vi "TopLevel.vi"() -> ()   [LabVIEW 2020]
uses:
  <vilib>/Averna/ProligentResultProcessor/ProligentResultProcessor.lvlibp/Datawarehouse/Datawarehouse.lvclass
panel:
  out "Passed":bool
  out "error out":errorcluster
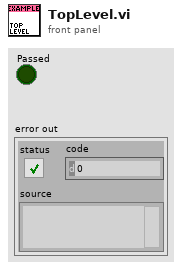
[diagram p1: front panel]
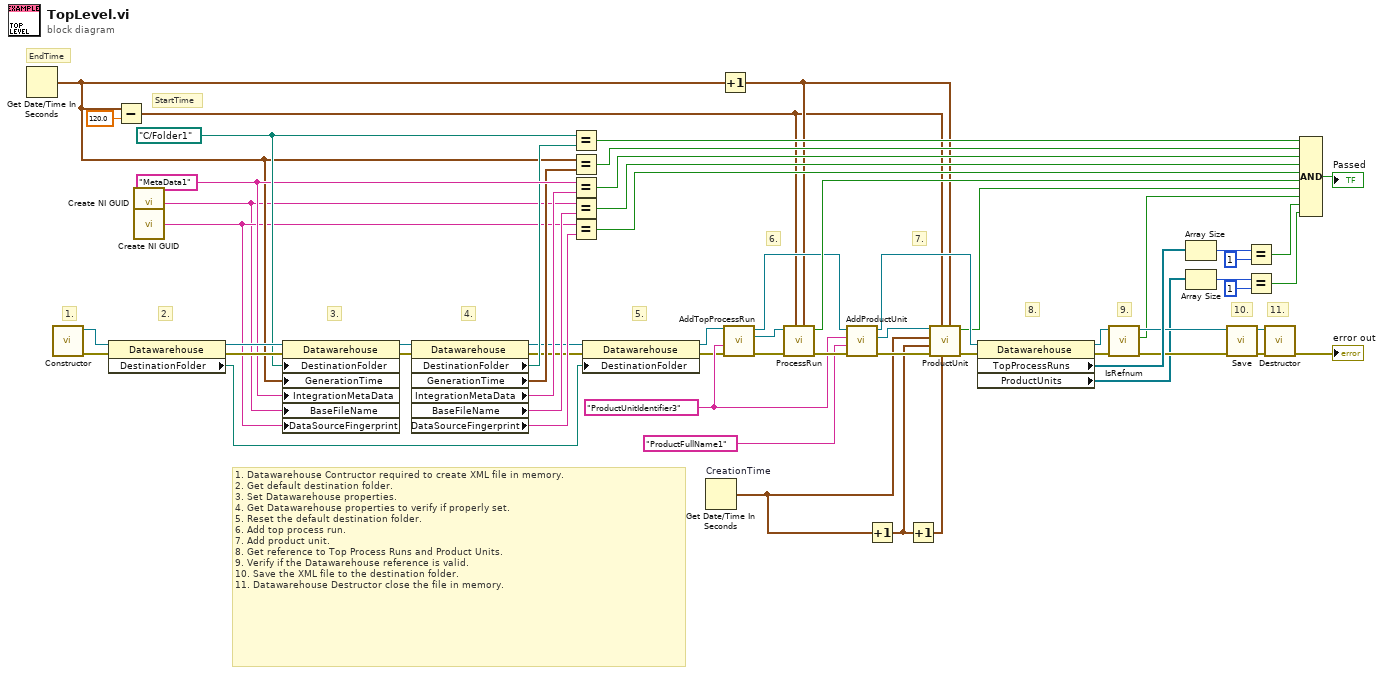
[diagram p0: block diagram]
diagram:
  w11 = "ProductUnitIdentifier3"
  w53 = "MetaData1"
  w54 = path "C:/Folder1"
  # "1. Datawarehouse Contructor required to create XML file in memory.\n2. Get default destination folder.\n3. Set Datawarehouse properties.\n4. Get Datawarehouse properties to verify if properly set.\n5. Reset the default destination folder.\n6. Add top process run.\n7. Add product unit.\n8. Get reference to Top Process Runs and Product Units.\n9. Verify if the Datawarehouse reference is valid.\n10. Save the XML file to the destination folder.\n11. Datawarehouse Destructor close the file in memory."
  # "11."
  # "10."
  # "9."
  # "8."
  # "7."
  # "6."
  # "5."
  # "4."
  # "3."
  # "2."
  # "1."
  # "EndTime"
  # "StartTime"
  n1 = Get Date/Time In Seconds ("Final Time")() -> (seconds since 1Jan1904=w10:timestamp)
  n2 = call <vilib>:"Constructor.vi"() -> ("error out"=w57:errorcluster, "Datawarehouse"=w58:refnum<class "Datawarehouse.lvclass">)  [unwired: 10 in]
  n3 = property class="Datawarehouse"(reference=w58, error in=w57) -> (reference out=w55:refnum<class "Datawarehouse.lvclass">, error out=w56:errorcluster, "DestinationFolder"=w32:path)
  n4 = Subtract(x=w10, y=120.0) -> (x-y=w9:timestamp)
  n5 = call <vilib>:"Create NI GUID.vi"() -> ("NI GUID"=w3:string)
  n6 = call <vilib>:"Create NI GUID.vi"() -> ("NI GUID"=w5:string)
  n7 = property class="Datawarehouse"(reference=w55, error in=w56, "DestinationFolder"=w54, "GenerationTime"=w10, "IntegrationMetaData"=w53, "BaseFileName"=w3, "DataSourceFingerprint"=w5) -> (reference out=w41:refnum<class "Datawarehouse.lvclass">, error out=w40:errorcluster)
  n8 = property class="Datawarehouse"(reference=w41, error in=w40) -> (reference out=w34:refnum<class "Datawarehouse.lvclass">, error out=w33:errorcluster, "DestinationFolder"=w39:path, "GenerationTime"=w38:timestamp, "IntegrationMetaData"=w37:string, "BaseFileName"=w36:string, "DataSourceFingerprint"=w35:string)
  n9 = Equal?(x=w54, y=w39) -> (x = y?=w52:bool)
  n10 = Equal?(x=w10, y=w38) -> (x = y?=w51:bool)
  n11 = Equal?(x=w53, y=w37) -> (x = y?=w50:bool)
  n12 = Equal?(x=w3, y=w36) -> (x = y?=w48:bool)
  n13 = Equal?(x=w5, y=w35) -> (x = y?=w47:bool)
  n14 = property class="Datawarehouse"(reference=w34, error in=w33, "DestinationFolder"=w32) -> (reference out=w1:refnum<class "Datawarehouse.lvclass">, error out=w2:errorcluster)
  n15 = Get Date/Time In Seconds "CreationTime"() -> (seconds since 1Jan1904=w8:timestamp)
  n16 = Increment(x=w10) -> (x+1=w14:timestamp)
  n17 = call <vilib>:"AddTopProcessRun.vi"("error in"=w2, "ProductUnitIdentifier"=w11, "Datawarehouse in"=w1) -> ("error out"=w46:errorcluster, "TopProcessRun"=w42:refnum<class "ProcessRun.lvclass">, "Datawarehouse out"=w17:refnum<class "Datawarehouse.lvclass">)  [unwired: 6 in]
  n18 = call "ProcessRun.vi"("EndTime"=w14, "StartTime"=w9, "error in"=w46, "ProcessRun"=w42) -> ("error out"=w19:errorcluster, "Passed"=w31:bool)  [unwired: 6 in]
  n19 = call <vilib>:"AddProductUnit.vi"("error in"=w19, "ProductFullName"="ProductFullName1", "ProductUnitIdentifier"=w11, "Datawarehouse in"=w17) -> ("error out"=w18:errorcluster, "ProductUnit"=w13:refnum<class "ProductUnit.lvclass">, "Datawarehouse out"=w16:refnum<class "Datawarehouse.lvclass">)  [unwired: 5 in]
  n20 = Increment(x=w8) -> (x+1=w7:timestamp)
  n21 = Increment(x=w7) -> (x+1=w6:timestamp)
  n22 = call "ProductUnit.vi"("EndTime"=w14, "ScrappedTime"=w6, "StartTime"=w9, "error in (no error)"=w18, "ManufacturingTime"=w7, "CreationTime"=w8, "ProductUnit in"=w13) -> ("error out"=w15:errorcluster, "Passed"=w4:bool)  [unwired: 3 in]
  n23 = property class="Datawarehouse"(reference=w16, error in=w15) -> (reference out=w27:refnum<class "Datawarehouse.lvclass">, error out=w45:errorcluster, "TopProcessRuns"=w44:refnum<class "ProcessRun.lvclass">[], "ProductUnits"=w20:refnum<class "ProductUnit.lvclass">[])
  n24 = call <vilib>:"IsRefnum.vi"("error in"=w45, "Datawarehouse in"=w27) -> ("error out"=w28:errorcluster, "IsRefnum"=w25:bool, "Datawarehouse out"=w26:refnum<class "Datawarehouse.lvclass">)  [unwired: 7 in]
  n25 = Array Size(array=w44) -> (size(s)=w43:i32)
  n26 = Array Size(array=w20) -> (size(s)=w22:i32)
  n27 = call <vilib>:"Save.vi"("error in"=w28, "Datawarehouse in"=w26) -> ("error out"=w59:errorcluster, "Datawarehouse out"=w60:refnum<class "Datawarehouse.lvclass">)  [unwired: 8 in]
  n28 = Equal?(x=w43, y=1) -> (x = y?=w30:bool)
  n29 = Equal?(x=w22, y=1) -> (x = y?=w21:bool)
  n30 = call <vilib>:"Destructor.vi"("error in"=w59, "Datawarehouse"=w60) -> ("error out"=→"error out":errorcluster)  [unwired: 9 in]
  n31 = Compound Arithmetic op=AND(w52, w51, w50, w48, w47, w31, w4, w25, w30, w21) -> (→"Passed":bool)
